vi "严格匹配.vi"(4 "搜索字符串":string, 5 "输入字符串":string) -> (0 "之后":string, 1 "搜索字符串":string, 2 "之前":string)   [LabVIEW 2020]
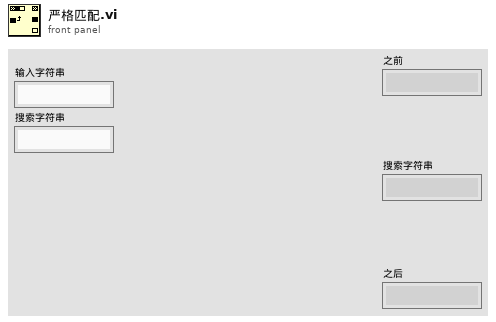
[diagram p1: front panel]
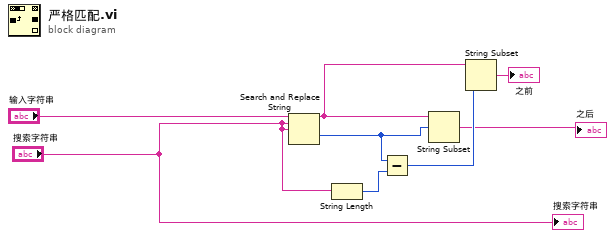
[diagram p0: block diagram]
diagram:
  n1 = Search and Replace String(input string="输入字符串", search string="搜索字符串", replace string="搜索字符串") -> (result string=w7:string, offset past replacement=w5:i32)  [unwired: 5 in, 2 out]
  n2 = String Length(string="搜索字符串") -> (length=w4:i32)
  n3 = Subtract(x=w5, y=w4) -> (x-y=w3:i32)
  n4 = String Subset(string=w7, offset (0)=w5) -> (substring=→"之后":string)  [unwired: 1 in]
  n5 = String Subset(string=w7, length (rest)=w3) -> (substring=→"之前":string)  [unwired: 1 in]
  "搜索字符串" <- "搜索字符串"
